vi "AV Write Array.vi"(8 "error in":errorcluster, 10 "Power AV":dbl[](array[numeric]), 11 "Power Actual Value in":refnum<class "Power Actual Value.lvclass">) -> (0 "error out":errorcluster, 3 "Power Actual Value out":refnum<class "Power Actual Value.lvclass">)   [LabVIEW 2023, in "Power Actual Value.lvclass"]
uses:
  Power Actual Value.lvclass
  Parents/Actual Value/Actual Value.lvclass
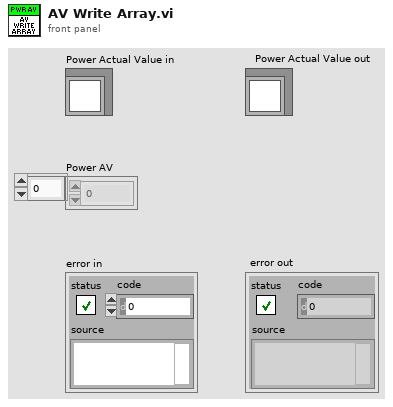
[diagram p1: front panel]
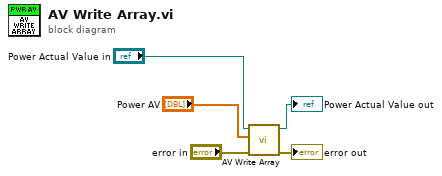
[diagram p0: block diagram]
diagram:
  n1 = call-parent "AV Write Array.vi"("error in"="error in", "Actual Value"="Power AV", "Actual Value in"="Power Actual Value in") -> ("error out"=→"error out":errorcluster, "Actual Value out"=→"Power Actual Value out":refnum<class "Power Actual Value.lvclass">)  [unwired: 7 in]
